vi "Post Block.vi"(8 "error in (no error)":errorcluster, 10 "Cluster":T1, 11 "Database.lvlib:Data Store.lvclass":refnum<class "Data Store.lvclass">) -> (0 "error out":errorcluster, 3 "Database.lvlib:Data Store.lvclass 2":refnum<class "Data Store.lvclass">)   [LabVIEW 2011, in "Database.lvlib" / "Data Store.lvclass"]
uses:
  Data Store.lvclass
  Block.ctl
  Data Store.lvclass/Data Store.ctl
  <vilib>/addons/database/NI_Database_API.lvlib
  Database.lvlib
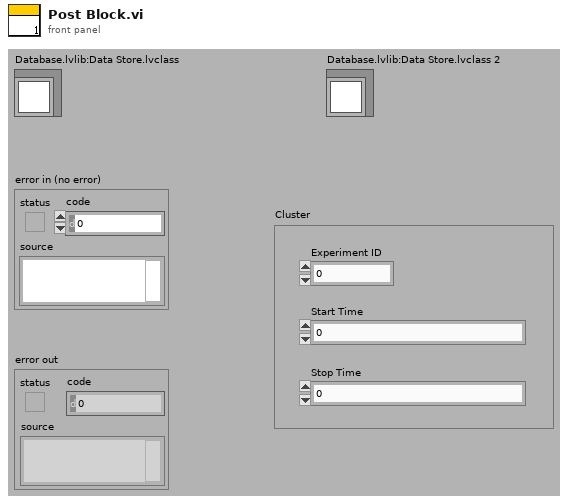
[diagram p1: front panel]
types:
  T1 = typedef "Database.lvlib/Block.ctl" = cluster{"Experiment ID":i32, "Start Time":u64, "Stop Time":u64}
  T2 = typedef "NI_Database_API.lvlib/Conn ObjectReference.ctl" = refnum<k1>
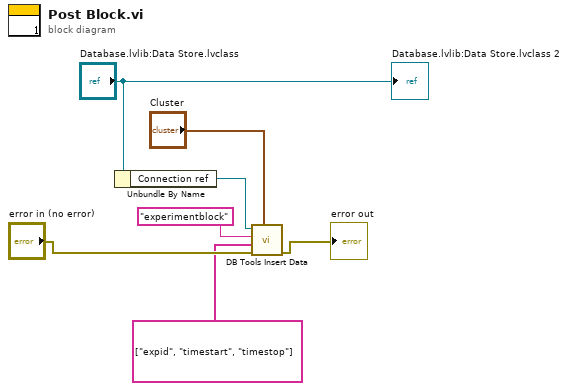
[diagram p0: block diagram]
diagram:
  n1 = Unbundle By Name("Database.lvlib:Data Store.lvclass") -> ("Connection ref"=w5:T2)
  n2 = call <vilib>:"DB Tools Insert Data.vi"("data"="Cluster", "error in (no error)"="error in (no error)", "columns"=string[] ["expid", "timestart", "timestop"], "table"="experimentblock", "connection reference"=w5) -> ("error out"=→"error out":errorcluster)  [unwired: 5 in, 1 out]
  "Database.lvlib:Data Store.lvclass 2" <- "Database.lvlib:Data Store.lvclass"
